vi "Configure Onboard Clock.vi"(0 "device session in":refnum<class "Device Session.lvclass">, 5 "reference clock source":T1, 7 "reference clock rate (Hz)":dbl=10000000.0 format="%#_6p", 9 "adc clock rate (Hz)":dbl=250000000.0 format="%#_6p", 11 "error in":errorcluster) -> (4 "device session out":refnum<class "Device Session.lvclass">, 6 "actual adc clock rate (Hz)":dbl=250000000.0 format="%#_6p", 8 "actual reference clock rate (Hz)":dbl format="%#_6p", 15 "error out":errorcluster)   [LabVIEW 2021, in "Device Session.lvclass"]
doc: "Configures the device to use an onboard clock as the source of the ADC clock. If a reference clock source is specified, this VI also phase locks the device to that clock.\n\n<B>Input Parameters</B>\n\n<B>device session in</B> is a reference to the Device Session object, which contains a session to each instrument design library used in this sample project. This parameter is obtained from the 'Open Session' VI.\n\n<B>reference clock source</B> specifies the source of the reference clock used to generate the onboard ADC Clock.\n\n'None' (default): specifies that no reference clock will be used.\n'Clock In': specifies that the clock source is the Clock In connector on the device front panel.\n'PXI Clock': specifies that the clock source is the clock signal from the PXI chassis.\n\n<B>reference clock rate (Hz)</B> specifies the input reference clock rate if the 'reference clock source' is Clock In. This parameter is ignored if the 'reference clock source' is None or PXI Clock.\n\n<B>adc clock rate (Hz)</B> specifies the clock rate to use for the onboard sample clock.\n\n<B>error in</B> describes error conditions that occur before this node runs. This input provides standard 'error in' functionality.\n\n<B>Output Parameters</B>\n\n<B>device session out</B> passes a reference to the session to the next VI.\n\n<B>actual adc clock rate (Hz)</B> returns the coerced value of the ADC clock rate.\n\n<B>actual reference clock rate (Hz)</B> returns the coerced reference clock rate.\n\n<B>error out</B> contains error information. This output provides standard 'error out' functionality."
uses:
  Device Session.lvclass
  <instrlib>/HSAI-RIO/Types/v1/Host/Typedefs/Reference Clock Source.ctl
  Device Session.lvclass/Device Session.ctl
  <instrlib>/HSAI-RIO/Config/Group A/v1/Host/Main/niHSAI Group A Config v1 Host.lvclass
  C:/Program Files (x86)/National Instruments/LabVIEW 2021/instr.lib/HSAI-RIO/Config/Interface/v1/Host/niHSAI Config v1 Host.lvclass
  <instrlib>/HSAI-RIO/Config/Interface/v1/Host/Protected/Configure ADC Clock For Onboard.vi
  <instrlib>/HSAI-RIO/Config/Interface/v1/Host/niHSAI Config v1 Host.lvclass
  C:/Program Files (x86)/National Instruments/LabVIEW 2021/instr.lib/HSAI-RIO/Config/Group A/v1/Host/Main/niHSAI Group A Config v1 Host.lvclass
  <instrlib>/HSAI-RIO/Types/v1/Host/niHSAI Types v1 Host.lvlib
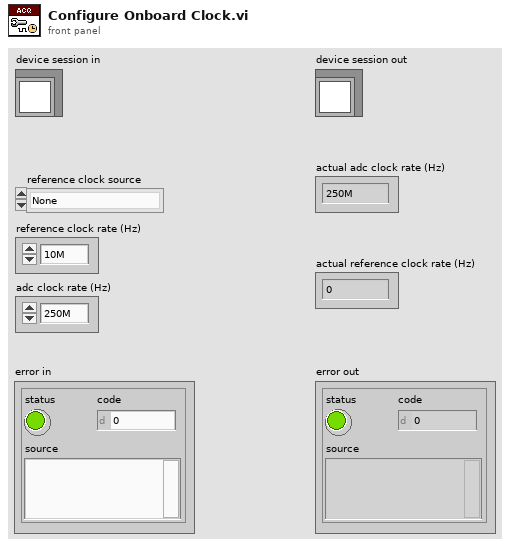
[diagram p1: front panel]
types:
  T1 = typedef "niHSAI Types v1 Host.lvlib/Reference Clock Source.ctl" = enum8{"None", "Clock In", "PXI Clock", "AUX 0 Clock In"}
  T2 = typedef "Device Session.lvclass/Device Session Object.ctl" = cluster{"fpga reference":T3, "reg bus":refnum<class "niInstr FIFO Register Bus v1 Host.lvclass">, "subsystem map":refnum<class "niInstr Subsystem Map v1 Host.lvclass">, "cal data":refnum<class "niHSAI Cal Data v1 Host.lvclass">, "config":refnum<class "niHSAI Group A Config v1 Host.lvclass">, "acquisition 0":refnum<class "niInstr Multirecord Acquisition v1 Host.lvclass">, "acquisition 1":refnum<class "niInstr Multirecord Acquisition v1 Host.lvclass">, "number of selected acq channels":u8, "selected acq channels":bool[], "number of channels":u32, "configured channels":bool[], "acq configuration":cluster{"number of samples":u64, "number of records":u64, "pretrigger samples":u64}, "actual channel configuration":T4[], "sample clock rate (Hz)":dbl, "scaling coefficients":T8[]}
  T3 = typedef "Device Session.lvclass/FPGA Refnum.ctl" = refnum<k20>
  T4 = typedef "niHSAI Types v1 Host.lvlib/Channel Configuration.ctl" = cluster{"channel":u32, "coupling":T5, "impedance":T6, "bandwidth":T7, "vertical range":dbl, "vertical offset":dbl}
  T5 = typedef "niHSAI Types v1 Host.lvlib/Coupling.ctl" = enum8{"Default", "DC", "AC"}
  T6 = typedef "niHSAI Types v1 Host.lvlib/Impedance.ctl" = enum8{"Default", "1 mega ohm", "50 ohm"}
  T7 = typedef "niHSAI Types v1 Host.lvlib/Bandwidth.ctl" = enum8{"Default", "Full Bandwidth", "Anti-alias Filter", "150 MHz"}
  T8 = typedef "niInstr Multirecord Acquisition v1 Host.lvclass/Scaling Coefficient.ctl" = cluster{"gain":dbl, "offset":dbl}
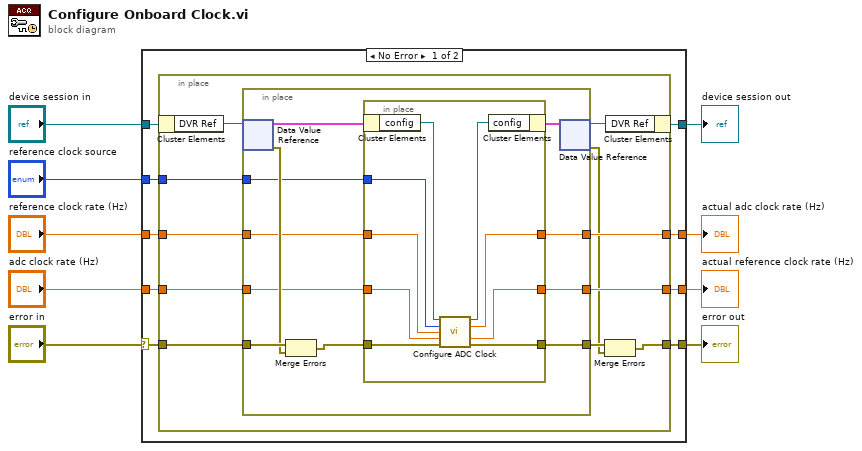
[diagram p0: block diagram]
diagram:
  n1 = case shown="No Error" "error in" {
    selector: "error in" -> [w18 w51]
    tunnel: "device session in" -> [w12 w50]
    tunnel: [w11 w50] -> w7
    tunnel: [w14 w51] -> w6
    tunnel: [w17 _] -> w4
    tunnel: [w16 _] -> w3
    tunnel: "reference clock rate (Hz)" -> [w15 _]
    tunnel: "reference clock source" -> [w13 _]
    tunnel: "adc clock rate (Hz)" -> [w10 _]
    frame No Error {
      n2 = in-place {
        in-place-border: w18 -> [w29]
        in-place-border: [w28] -> w17
        in-place-border: [w26] -> w16
        in-place-border: w15 -> [w25]
        in-place-border: [w20] -> w14
        in-place-border: w13 -> [w23]
        in-place-border: w10 -> [w19]
        n3 = in-place-cluster #1(w12) -> ("DVR Ref"=w22:refnum<data-value>)
        n4 = in-place {
          in-place-border: w29 -> [w39]
          in-place-border: [w33] -> w28
          in-place-border: [w40] -> w27
          in-place-border: [w32] -> w26
          in-place-border: w25 -> [w35]
          in-place-border: w23 -> [w34]
          in-place-border: w19 -> [w30]
          n5 = in-place-dvr #2(w22) -> (w36:T2, w38:errorcluster)
          n6 = Merge Errors(w39, w38) -> (w37:errorcluster)
          n7 = in-place {
            in-place-border: [w49] -> w40
            in-place-border: w37 -> [w48]
            in-place-border: w35 -> [w47]
            in-place-border: w34 -> [w46]
            in-place-border: [w43] -> w33
            in-place-border: [w44] -> w32
            in-place-border: w30 -> [w41]
            n8 = in-place-cluster #3(w36) -> ("config"=w45:refnum<class "niHSAI Group A Config v1 Host.lvclass">)
            n9 = call-poly <instrlib>:"Configure ADC Clock.vi"("session in"=w45, "reference clock source"=w46, "reference clock rate (Hz)"=w47, "adc clock rate (Hz)"=w41, "error in"=w48) -> ("session out"=w42:refnum<class "niHSAI Group A Config v1 Host.lvclass">, "actual adc clock rate (Hz)"=w43:dbl, "actual reference clock rate (Hz)"=w44:dbl, "error out"=w49:errorcluster)  [unwired: 6 in, 1 out]
            n10 = in-place-cluster #3("config"=w42) -> (w31:T2)
          }
          n11 = in-place-dvr #2(w31) -> (w21:refnum<data-value>, w24:errorcluster)
        }
        n12 = Merge Errors(w27, w24) -> (w20:errorcluster)
        n13 = in-place-cluster #1("DVR Ref"=w21) -> (w11:refnum<class "Device Session.lvclass">)
      }
    }
    frame Error {
    }
  }
  "error out" <- w6
  "device session out" <- w7
  "actual adc clock rate (Hz)" <- w4
  "actual reference clock rate (Hz)" <- w3
